vi "Untitled 4.vi"   [LabVIEW 2020]
uses:
  Advanced Assertions.lvlib
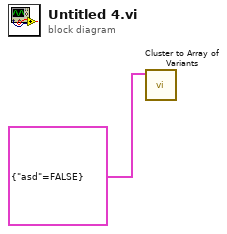
[diagram p0: block diagram]
diagram:
  n1 = call "Cluster to Array of Variants.vi"("Expected Cluster"=cluster{"asd":bool} {"asd"=FALSE}) -> ()  [unwired: 9 in, 2 out]
